vi "Write Trace.vi"(4 "Error In":errorcluster, 6 "Trace Data":string, 7 "Trace Point Name":string) -> (0 "Error Out":errorcluster)   [LabVIEW 2014, in "Debugging.lvlib"]
uses:
  Debugging.lvlib
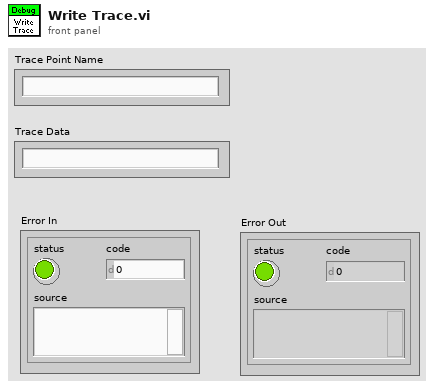
[diagram p1: front panel]
types:
  T1 = enum16{"open", "replace", "create", "open or create", "replace or create", "replace or create with confirmation"}
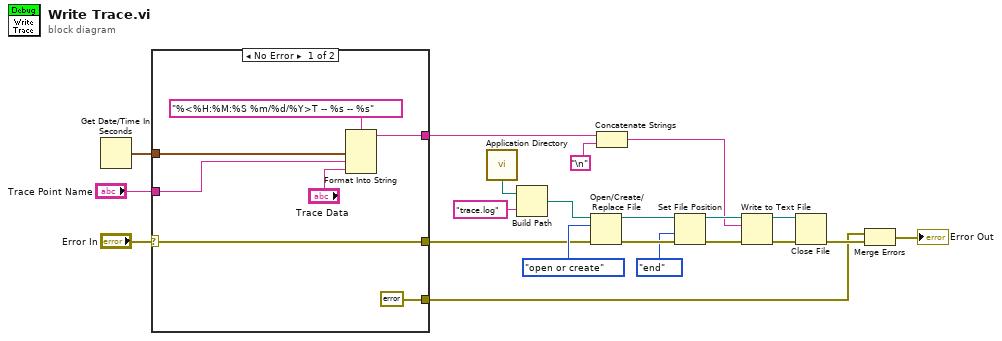
[diagram p0: block diagram]
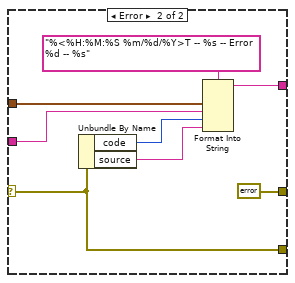
[diagram p2: hidden frame]
diagram:
  n1 = Get Date/Time In Seconds() -> (seconds since 1Jan1904=w4:timestamp)
  n2 = case shown="No Error" "Error In" {
    selector: "Error In" -> [w28 w31]
    tunnel: [w28 errorcluster {"status"=FALSE, "code"=0, "source"=""} ("error IO")] -> w9
    tunnel: [errorcluster {"status"=FALSE, "code"=0, "source"=""} ("error IO") w31] -> w6
    tunnel: [w25 w32] -> w5
    tunnel: w4 -> [w23 w34]
    tunnel: "Trace Point Name" -> [w22 w33]
    frame No Error {
      n3 = Format Into String(format string="%<%H:%M:%S %m/%d/%Y>T -- %s -- %s", w23, w22, "Trace Data") -> (resulting string=w25:string)  [unwired: 2 in, 1 out]
    }
    frame Error {
      n4 = Unbundle By Name(w31) -> ("code"=w30:i32, "source"=w29:string)
      n5 = Format Into String(format string="%<%H:%M:%S %m/%d/%Y>T -- %s -- Error %d -- %s", w34, w33, w30, w29) -> (resulting string=w32:string)  [unwired: 2 in, 1 out]
    }
  }
  n6 = call <vilib>:"Application Directory.vi"() -> ("Application Directory"=w21:path)
  n7 = Build Path(base path=w21, name or relative path="trace.log") -> (appended path=w19:path)
  n8 = Open/Create/Replace File(file path (use dialog)=w19, error in=w9, operation (0:open)=T1."open or create") -> (refnum out=w16:refnum<file>, error out=w17:errorcluster)  [unwired: 3 in, 1 out]
  n9 = Concatenate Strings(w5, "\n") -> (w2:string)
  n10 = Set File Position(refnum=w16, from (0:start)=enum16{"start", "end", "current"}."end", error in=w17) -> (refnum out=w13:refnum<file>, error out=w14:errorcluster)  [unwired: 1 in]
  n11 = Write to Text File(file (use dialog)=w13, text=w2, error in=w14) -> (refnum out=w12:refnum<file>, error out=w11:errorcluster)  [unwired: 1 in, 1 out]
  n12 = Close File(refnum=w12, error in=w11) -> (error out=w10:errorcluster)  [unwired: 1 out]
  n13 = Merge Errors(w6, w10) -> (→"Error Out":errorcluster)
